vi "Alarma_IEEE45_G01.vi"(8 "error in (no error)":errorcluster) -> (0 "error out":errorcluster)   [LabVIEW 2018]
uses:
  Controls/Cluster_Alarmas_IEEE45.ctl
  <vilib>/RAFA Solutions/Harmony UI Controls Kit/Boolean/Round Led.ctl
  <vilib>/addons/database/Connection.llb/DB Tools Open Connec (Path).vi
  Global/Demo.vi
  Global/Alarmas_indicadores-LED.vi
  Global/AlarmasGlobal.vi
  <vilib>/addons/database/NI_Database_API.lvlib
  <vilib>/RAFA Solutions/Harmony UI Controls Kit/Flat UI Design.lvlib
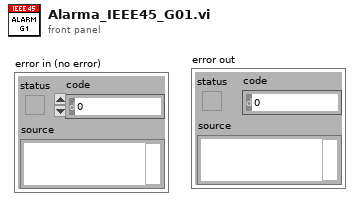
[diagram p1: front panel]
types:
  T1 = typedef "NI_Database_API.lvlib/Conn ObjectReference.ctl" = refnum<k1>
  T2 = typedef "Cluster_Alarmas_IEEE45.ctl" = cluster{"V1_V2 (V) ":cluster{dbl, dbl, dbl}, "Mod_V1_V2":dbl, "alarma 1":T3, "Mod_V2_V3":dbl, "alarma 2":T3, "Mod_V3_V1":dbl, "alarma 3":T3, "Mod_Frec":dbl, "alarma 4":T3, "V2_V3 (V)":cluster{dbl, dbl, dbl}, "V3_V1 (V)":cluster{dbl, dbl, dbl}, "Frecuencia (Hz)":cluster{dbl, dbl, dbl}, "AVG VL_VL (V)":cluster{dbl, dbl, dbl}, "alarm 5":bool, "alarm 6":bool, "alarm 7":bool, "alarm 8":bool, "alarm 9":bool}
  T3 = typedef "Flat UI Design.lvlib/Round Led.ctl" = bool
  T4 = typedef "VIF_cluster.ctl" = cluster{"VL_VL":cluster{"V1_V2":sgl, "V2_V3":sgl, "V3_V1":sgl, "Avg_VL_VL":sgl}, "IL_IL":cluster{"I1":sgl, "I2":sgl, "I3":sgl, "Avg_Amps":sgl}, "Frecuency":sgl, "Avg_Frecuency":sgl}
  T5 = cluster{"V1_V2":sgl, "V2_V3":sgl, "V3_V1":sgl, "Avg_VL_VL":sgl}
  T6 = cluster{"Mod_V1_V2":sgl, "Mod_V2_V3":sgl, "Mod_V3_V1":sgl, "alarma 1":bool, "alarma 2":bool, "alarma 3":bool}
  T7 = cluster{"alarm 5":bool, "alarm 6":bool, "alarm 7":bool, "alarm 8":bool, "alarm 9":bool}
  T8 = cluster{"Frecuency Modulation (%)":sgl, "alarma":bool}
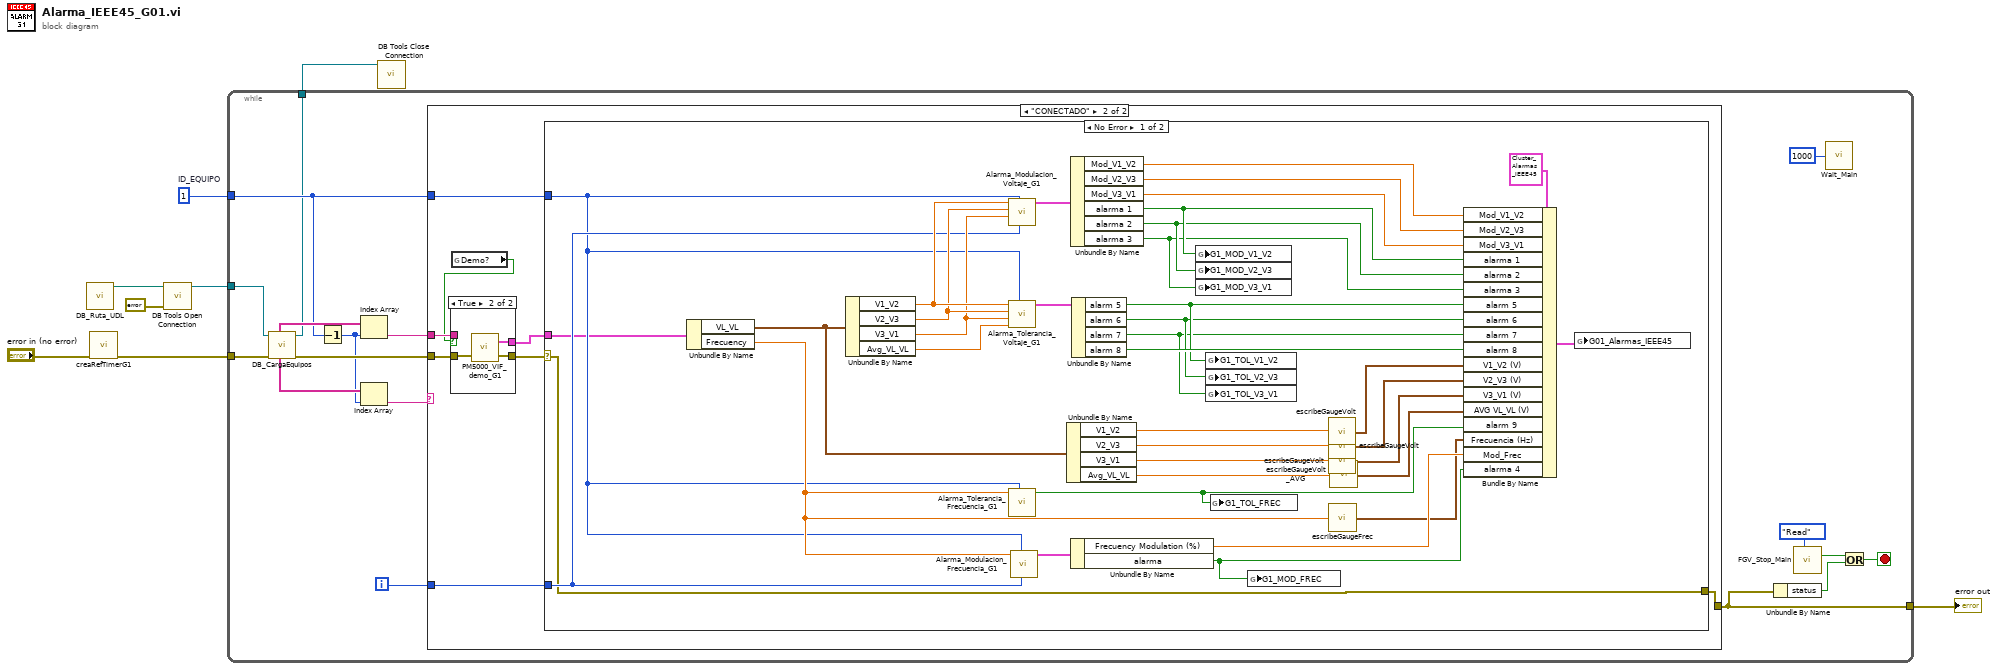
[diagram p0: block diagram]
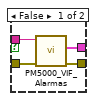
[diagram p3: hidden frame]
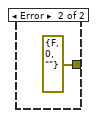
[diagram p4: hidden frame]
diagram:
  w6 = 1  # ID_EQUIPO
  n1 = call "DB_Ruta_UDL.vi"() -> ("UDL ruta"=w3:path)  [unwired: 11 in]
  n2 = call "creaRefTimerG1.vi"("error in (no error)"="error in (no error)") -> ("error out"=w7:errorcluster)  [unwired: 10 in]
  n3 = call-poly <vilib>:"DB Tools Open Connection.vi"("error in (no error)"=errorcluster {"status"=FALSE, "code"=0, "source"=""}, "connection information"=w3) -> ("connection reference"=w2:T1)  [unwired: 6 in, 1 out]
  n4 = while {
    tunnel: w7 -> [w15]
    tunnel: w6 -> [w16]
    tunnel: [w19] -> w5
    tunnel: w2 -> [w17]
    tunnel: [w14] -> w1
    i -> [w23]
    stop <- w22 stop-if-true
    n5 = call "DB_CargaEquipos.vi"("error in (no error)"=w15, "db in"=w17) -> ("error out"=w13:errorcluster, "db out"=w14:T1, "ESTADO_EQUIPO"=w11:string[], "IP_EQUIPOS"=w18:string[])  [unwired: 2 in, 4 out]
    n6 = Decrement(x=w16) -> (x-1=w10:i32)
    n7 = Index Array(array=w18, index=w10) -> (element=w12:string)
    n8 = Index Array(array=w11, index=w10) -> (element=w9:string)
    n9 = case shown="\"CONECTADO\"" w9 {
      tunnel: w23 -> [_ w33]
      tunnel: [_ w32] -> w19
      tunnel: w16 -> [_ w31]
      tunnel: w13 -> [_ w30]
      tunnel: w12 -> [_ w28]
      frame Default {
      }
      frame "CONECTADO" {
        n10 = global read "Demo.vi" "Demo?"() -> (w26:bool)
        n11 = case shown="True" w26 {
          tunnel: w30 -> [w37 w38]
          tunnel: [w36 w39] -> w29
          tunnel: w28 -> [w35 _]
          tunnel: [w34 w40] -> w27
          frame False {
            n12 = call "PM5000_VIF_Alarmas.vi"("error in"=w37, "Network Path"=w35) -> ("error out"=w36:errorcluster, "output cluster"=w34:T4)  [unwired: 7 in, 1 out]
          }
          frame True {
            n13 = call "PM5000_VIF_demo_G1.vi"("error in (no error)"=w38) -> ("error out"=w39:errorcluster, "VIF_cluster"=w40:T4)  [unwired: 1 in]
          }
        }
        n14 = case shown="No Error" w29 {
          selector: w29 -> [w44 _]
          tunnel: w33 -> [w60 _]
          tunnel: w31 -> [w45 _]
          tunnel: [w44 errorcluster {"status"=FALSE, "code"=0, "source"=""} ("error out")] -> w32
          tunnel: w27 -> [w43 _]
          frame No Error {
            n15 = Unbundle By Name(w43) -> ("VL_VL"=w69:T5, "Frecuency"=w59:sgl)
            n16 = Unbundle By Name(w69) -> ("V1_V2"=w77:sgl, "V2_V3"=w76:sgl, "V3_V1"=w75:sgl, "Avg_VL_VL"=w74:sgl)
            n17 = call "Alarma_Modulacion_Voltaje_G1.vi"("# iteration"=w60, "ID_EQUIPO"=w45, "V3_V1"=w75, "V2_V3"=w76, "V1_V2"=w77) -> ("Alarma_Mod_Volt out"=w73:T6)  [unwired: 6 in]
            n18 = call "Alarma_Tolerancia_Voltaje_G1.vi"("ID_EQUIPO"=w45, "AVG_VL_VL"=w74, "V3_V1"=w75, "V2_V3"=w76, "V1_V2"=w77) -> ("alarm out"=w57:T7)  [unwired: 6 in]
            n19 = call "Alarma_Tolerancia_Frecuencia_G1.vi"("ID_EQUIPO"=w45, "Señal in"=w59) -> ("alarm"=w47:bool)  [unwired: 9 in]
            n20 = call "Alarma_Modulacion_Frecuencia_G1.vi"("# iteration"=w60, "ID_EQUIPO"=w45, "Frecuencia"=w59) -> ("Mod_Frec out"=w58:T8)  [unwired: 8 in]
            n21 = Unbundle By Name(w69) -> ("V1_V2"=w68:sgl, "V2_V3"=w67:sgl, "V3_V1"=w66:sgl, "Avg_VL_VL"=w63:sgl)
            n22 = Unbundle By Name(w73) -> ("Mod_V1_V2"=w72:sgl, "Mod_V2_V3"=w71:sgl, "Mod_V3_V1"=w70:sgl, "alarma 1"=w54:bool, "alarma 2"=w53:bool, "alarma 3"=w52:bool)
            n23 = Unbundle By Name(w58) -> ("Frecuency Modulation (%)"=w61:sgl, "alarma"=w46:bool)
            n24 = Unbundle By Name(w57) -> ("alarm 5"=w51:bool, "alarm 6"=w50:bool, "alarm 7"=w49:bool, "alarm 8"=w56:bool)
            n25 = global write "Alarmas_indicadores-LED.vi" "G1_MOD_V1_V2"(w54) -> ()
            n26 = global write "Alarmas_indicadores-LED.vi" "G1_MOD_V2_V3"(w53) -> ()
            n27 = global write "Alarmas_indicadores-LED.vi" "G1_MOD_V3_V1"(w52) -> ()
            n28 = global write "Alarmas_indicadores-LED.vi" "G1_TOL_V1_V2"(w51) -> ()
            n29 = global write "Alarmas_indicadores-LED.vi" "G1_TOL_V2_V3"(w50) -> ()
            n30 = global write "Alarmas_indicadores-LED.vi" "G1_TOL_V3_V1"(w49) -> ()
            n31 = global write "Alarmas_indicadores-LED.vi" "G1_TOL_FREC"(w47) -> ()
            n32 = global write "Alarmas_indicadores-LED.vi" "G1_MOD_FREC"(w46) -> ()
            n33 = call "escribeGaugeVolt.vi"("Vin"=w68) -> ("V_V out"=w65:cluster{"Max":sgl, "Vin":sgl, "Min":sgl})
            n34 = call "escribeGaugeVolt.vi"("Vin"=w67) -> ("V_V out"=w48:cluster{"Max":sgl, "Vin":sgl, "Min":sgl})
            n35 = call "escribeGaugeVolt.vi"("Vin"=w66) -> ("V_V out"=w64:cluster{"Max":sgl, "Vin":sgl, "Min":sgl})
            n36 = call "escribeGaugeFrec.vi"("Fin"=w59) -> ("Frec out"=w55:cluster{"Max":sgl, "Vin":sgl, "Min":sgl})
            n37 = call "escribeGaugeVolt_AVG.vi"("Vin"=w63) -> ("V_V out"=w62:cluster{"Max":sgl, "Vin":sgl, "Min":sgl})
            n38 = Bundle By Name(cluster=T2 {"V1_V2 (V) "={0.0, 17.0, 16.662651515468255}, "Mod_V1_V2"=0.0, "alarma 1"=FALSE, "Mod_V2_V3"=0.0, "alarma 2"=FALSE, "Mod_V3_V1"=0.0, "alarma 3"=FALSE, "Mod_Frec"=0.0, "alarma 4"=FALSE, "V2_V3 (V)"={0.0, 17.0, 16.662651515468255}, "V3_V1 (V)"={0.0, 17.0, 16.662651515468255}, "Frecuencia (Hz)"={0.0, 17.0, 16.662651515468255}, "AVG VL_VL (V)"={0.0, 17.0, 16.662651515468255}, "alarm 5"=FALSE, "alarm 6"=FALSE, "alarm 7"=FALSE, "alarm 8"=FALSE, "alarm 9"=FALSE} ("G01_Alarmas_IEEE45"), "Mod_V1_V2"=w72, "Mod_V2_V3"=w71, "Mod_V3_V1"=w70, "alarma 1"=w54, "alarma 2"=w53, "alarma 3"=w52, "alarm 5"=w51, "alarm 6"=w50, "alarm 7"=w49, "alarm 8"=w56, "V1_V2 (V)"=w65, "V2_V3 (V)"=w48, "V3_V1 (V)"=w64, "AVG VL_VL (V)"=w62, "alarm 9"=w47, "Frecuencia (Hz)"=w55, "Mod_Frec"=w61, "alarma 4"=w46) -> (w41:T2)
            n39 = global write "AlarmasGlobal.vi" "G01_Alarmas_IEEE45"(w41) -> ()
          }
          frame Error {
          }
        }
      }
    }
    n40 = Unbundle By Name(w19) -> ("status"=w20:bool)
    n41 = call "FGV_Stop_Main.vi"("Action"=enum16{"Read", "Write"}."Read") -> ("Var Out"=w21:bool)  [unwired: 9 in, 1 out]
    n42 = call "Wait_Main.vi"("Wait time (msec)"=u32 1000 ("delay (ms)")) -> ()  [unwired: 5 in]
    n43 = Or(x=w21, y=w20) -> (x .or. y?=w22:bool)
  }
  "error out" <- w5
  n44 = call <vilib>:"DB Tools Close Connection.vi"("connection reference"=w1) -> ()  [unwired: 6 in, 1 out]
